vi "Check image quality.vi"(8 "error in (no error)":errorcluster, 11 "Retiga in":refnum<class "Retiga.lvclass">) -> (0 "error out":errorcluster, 2 "QC passed?":bool, 3 "Retiga out":refnum<class "Retiga.lvclass">)   [LabVIEW 2012, in "Retiga.lvclass"]
uses:
  Retiga.lvclass
  Retiga.lvclass/Retiga.ctl
  <vilib>/vision/NI_Vision_Development_Module.lvlib
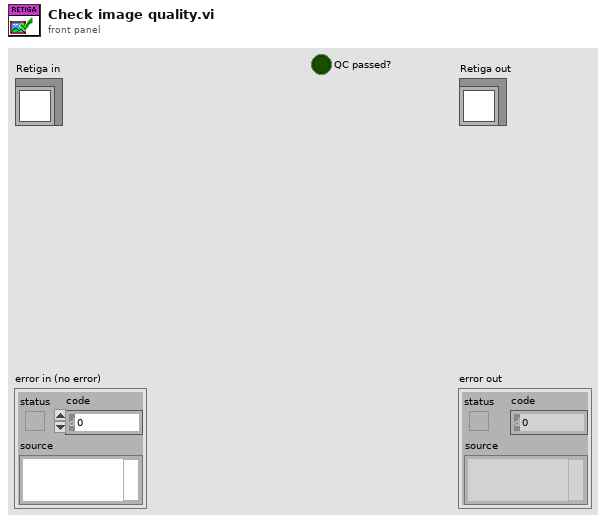
[diagram p1: front panel]
types:
  T1 = typedef "IMAQ Image.ctl" = refnum<image>
  T2 = cluster{"histogram":u32[], "Minimal Value":sgl, "Maximal Value":sgl, "Starting Value":sgl, "Interval Width":sgl, "Mean Value":sgl, "Standard  Variation":sgl, "Area (pixels)":i32}
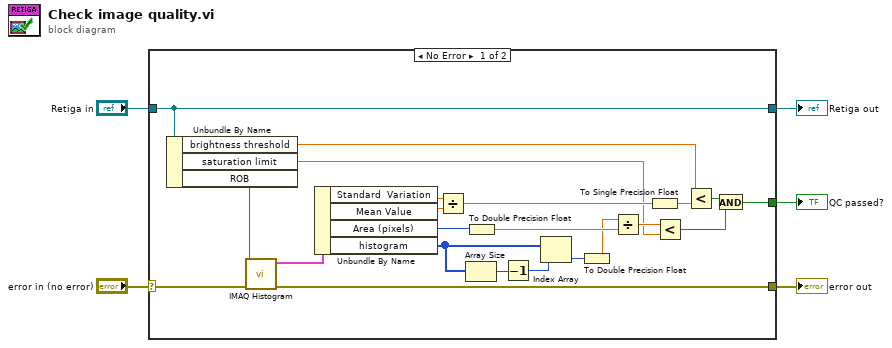
[diagram p0: block diagram]
diagram:
  n1 = case shown="No Error" "error in (no error)" {
    selector: "error in (no error)" -> [w8 w29]
    tunnel: [w7 w29] -> w4
    tunnel: [w12 w28] -> w2
    tunnel: "Retiga in" -> [w12 w28]
    tunnel: [w6 _] -> w1
    frame No Error {
      n2 = Unbundle By Name(w12) -> ("brightness threshold"=w10:sgl, "saturation limit"=w9:dbl, "ROB"=w11:T1)
      n3 = call "IMAQ Histogram"("error in (no error)"=w8, "Image"=w11) -> ("error out"=w7:errorcluster, "Histogram Report"=w26:T2)  [unwired: 8 in]
      n4 = Unbundle By Name(w26) -> ("Standard  Variation"=w25:sgl, "Mean Value"=w24:sgl, "Area (pixels)"=w19:i32, "histogram"=w22:u32[])
      n5 = Divide(x=w25, y=w24) -> (x/y=w23:sgl)
      n6 = Array Size(array=w22) -> (size(s)=w21:i32)
      n7 = To Double Precision Float(number=w19) -> (double precision float=w17:dbl)
      n8 = Decrement(x=w21) -> (x-1=w20:i32)
      n9 = Index Array(array=w22, index=w20) -> (element=w18:u32)
      n10 = To Double Precision Float(number=w18) -> (double precision float=w15:dbl)
      n11 = Divide(x=w15, y=w17) -> (x/y=w16:dbl)
      n12 = To Single Precision Float(number=w23) -> (single precision float=w27:sgl)
      n13 = Less?(x=w16, y=w9) -> (x < y?=w14:bool)
      n14 = Less?(x=w10, y=w27) -> (x < y?=w13:bool)
      n15 = And(x=w13, y=w14) -> (x .and. y?=w6:bool)
    }
    frame Error {
    }
  }
  "error out" <- w4
  "Retiga out" <- w2
  "QC passed?" <- w1
